vi "Create Contructor VIs.vi"   [LabVIEW 2015]
types:
  T1 = typedef "LVPositionTypeDef.ctl" = cluster{"Left":i32, "Top":i32}
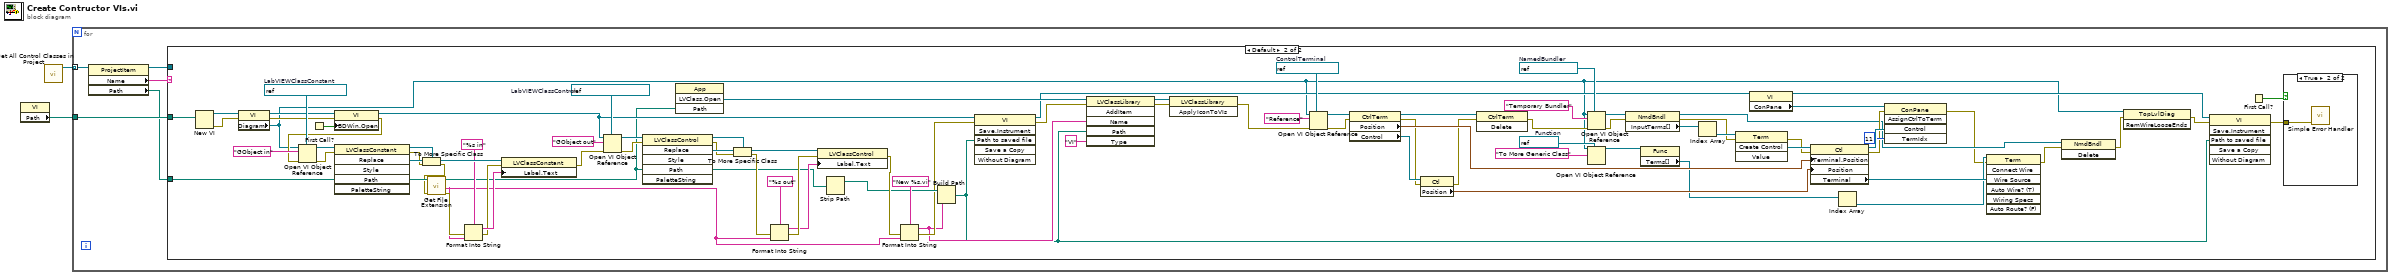
[diagram p0: block diagram]
diagram:
  n1 = property class="VI"() -> ("Path"=w1:path)  [unwired: 2 in, 2 out]
  n2 = call "Get All Control Classes in Project.vi"() -> ("All Control Classes"=w2:refnum<vi>[])  [unwired: 11 in]
  n3 = for {
    tunnel: w2 -> [w7] mode=indexing
    tunnel: w1 -> [w4]
    n4 = property class="ProjectItem"(reference=w7) -> (reference out=w5:refnum<vi>, "Name"=w6:string, "Path"=w3:path)  [unwired: 1 in, 1 out]
    n5 = case shown="Default" w6 {
      tunnel: w5 -> [_ _]
      tunnel: w4 -> [_ w96]
      tunnel: w3 -> [_ w79]
      frame "GObject.lvclass", "Generic.lvclass" {
      }
      frame Default {
        w18 = refnum<vi> refnum  # Function
        w43 = refnum<vi> refnum  # ControlTerminal
        w47 = refnum<vi> refnum  # NamedBundler
        w91 = refnum<vi> refnum  # LabVIEWClassControl
        w93 = refnum<vi> refnum  # LabVIEWClassConstant
        n6 = New VI(10:w96) -> (0:w86:errorcluster, 3:w95:refnum<vi>)  [unwired: 6 in]
        n7 = property class="VI"(reference=w95, error in=w86) -> (reference out=w85:refnum<vi>, error out=w84:errorcluster, "Diagram"=w10:refnum<vi>)
        n8 = First Call?() -> (First Call?: T/F=w22:bool)
        n9 = property class="VI"(reference=w85, error in=w84, "BDWin.Open"=w22) -> (reference out=w62:refnum<vi>, error out=w83:errorcluster)
        n10 = Open VI Object Reference(7:w93, 8:w83, 10:"GObject in" ("name/order"), 11:w10) -> (0:w87:errorcluster, 3:w92:refnum<vi>)
        n11 = invoke class="LVClassConstant" method="Replace"(reference=w92, error in=w87, "Path"=w79) -> (reference out=w80:refnum<vi>, error out=w74:errorcluster, "Replace"=w82:refnum<vi>)  [unwired: 3 in, 3 out]
        n12 = To More Specific Class(target class=w80, reference=w82, error in=w74) -> (specific class reference=w81:refnum<vi>, error out=w73:errorcluster)
        n13 = call <vilib>:"Get File Extension.vi"("error in (no error)"=w73, "file"=w79) -> ("error out"=w72:errorcluster, "filename without extension"=w59:string, "dup file"=w61:path)  [unwired: 5 in, 2 out]
        n14 = Format Into String(format string="%s in", error in=w72, w59) -> (resulting string=w77:string, error out=w71:errorcluster)  [unwired: 1 in]
        n15 = property class="LVClassConstant"(reference=w81, error in=w71, "Label.Text"=w77) -> (error out=w70:errorcluster)  [unwired: 1 out]
        n16 = Open VI Object Reference(7:w91, 8:w70, 10:"GObject out" ("name/order"), 11:w62) -> (0:w88:errorcluster, 3:w89:refnum<vi>)
        n17 = invoke class="LVClassControl" method="Replace"(reference=w89, error in=w88, "Path"=w61) -> (reference out=w75:refnum<vi>, error out=w69:errorcluster, "Replace"=w76:refnum<vi>)  [unwired: 3 in, 3 out]
        n18 = invoke class="App" method="LVClass.Open"("Path"=w61) -> ("LVClass.Open"=w63:refnum<vi>)  [unwired: 3 in, 3 out]
        n19 = To More Specific Class(target class=w75, reference=w76, error in=w69) -> (specific class reference=w66:refnum<vi>, error out=w68:errorcluster)
        n20 = Format Into String(format string="%s out", error in=w68, w59) -> (resulting string=w64:string, error out=w65:errorcluster)  [unwired: 1 in]
        n21 = property class="LVClassControl"(reference=w66, error in=w65, "Label.Text"=w64) -> (error out=w58:errorcluster)  [unwired: 1 out]
        n22 = Strip Path(path=w61) -> (stripped path=w57:path)  [unwired: 1 out]
        n23 = Format Into String(format string="New %s.vi", error in=w58, w59) -> (resulting string=w55:string, error out=w56:errorcluster)  [unwired: 1 in]
        n24 = Build Path(base path=w57, name or relative path=w55) -> (appended path=w50:path)
        n25 = invoke class="VI" method="Save.Instrument"(reference=w62, error in=w56, "Path to saved file"=w50) -> (reference out=w28:refnum<vi>, error out=w54:errorcluster)  [unwired: 3 in, 4 out]
        n26 = invoke class="LVClassLibrary" method="AddItem"(reference=w63, error in=w54, "Name"=w55, "Path"=w50, "Type"="VI") -> (reference out=w52:refnum<vi>, error out=w51:errorcluster)  [unwired: 1 in, 4 out]
        n27 = invoke class="LVClassLibrary" method="ApplyIconToVIs"(reference=w52, error in=w51) -> (error out=w42:errorcluster)  [unwired: 1 in, 2 out]
        n28 = Open VI Object Reference(7:w43, 8:w42, 10:"Reference" ("name/order"), 11:w10) -> (0:w40:errorcluster, 3:w41:refnum<vi>)
        n29 = property class="CtrlTerm"(reference=w41, error in=w40) -> (reference out=w35:refnum<vi>, error out=w31:errorcluster, "Position"=w33:T1, "Control"=w32:refnum<vi>)
        n30 = property class="Ctl"(reference=w32, error in=w31) -> (error out=w30:errorcluster, "Position"=w29:T1)  [unwired: 1 out]
        n31 = invoke class="CtrlTerm" method="Delete"(reference=w35, error in=w30) -> (error out=w34:errorcluster)  [unwired: 1 in, 2 out]
        n32 = Open VI Object Reference(7:w47, 8:w34, 10:"Temporary Bundler" ("name/order"), 11:w10) -> (0:w38:errorcluster, 3:w48:refnum<vi>)
        n33 = Open VI Object Reference(7:w18, 10:"To More Generic Class" ("name/order"), 11:w10) -> (3:w16:refnum<vi>)  [unwired: 1 in, 1 out]
        n34 = property class="NmdBndl"(reference=w48, error in=w38) -> (reference out=w13:refnum<vi>, error out=w37:errorcluster, "InputTerms[]"=w46:refnum<vi>[])
        n35 = property class="Func"(reference=w16) -> ("Terms[]"=w15:refnum<vi>[])  [unwired: 1 in, 2 out]
        n36 = Index Array(array=w46) -> (element=w45:refnum<vi>)  [unwired: 1 in]
        n37 = invoke class="Term" method="Create Control"(reference=w45, error in=w37) -> (error out=w36:errorcluster, "Create Control"=w39:refnum<vi>)  [unwired: 2 in, 2 out]
        n38 = property class="VI"(reference=w28) -> (reference out=w27:refnum<vi>, "ConPane"=w26:refnum<vi>)  [unwired: 1 in, 1 out]
        n39 = property class="Ctl"(reference=w39, error in=w36, "Terminal.Position"=w33, "Position"=w29) -> (reference out=w25:refnum<vi>, error out=w23:errorcluster, "Terminal"=w19:refnum<vi>)
        n40 = Index Array(array=w15) -> (element=w14:refnum<vi>)  [unwired: 1 in]
        n41 = invoke class="ConPane" method="AssignCtrlToTerm"(reference=w26, error in=w23, "Control"=w25, "TermIdx"=u32 11 ("Terminal Index")) -> (error out=w11:errorcluster)  [unwired: 1 in, 4 out]
        n42 = invoke class="Term" method="Connect Wire"(reference=w14, error in=w11, "Wire Source"=w19) -> (error out=w12:errorcluster)  [unwired: 4 in, 6 out]
        n43 = invoke class="NmdBndl" method="Delete"(reference=w13, error in=w12) -> (error out=w9:errorcluster)  [unwired: 1 in, 2 out]
        n44 = invoke class="TopLvlDiag" method="RemWireLooseEnds"(reference=w10, error in=w9) -> (error out=w8:errorcluster)  [unwired: 1 in, 2 out]
        n45 = invoke class="VI" method="Save.Instrument"(reference=w27, error in=w8, "Path to saved file"=w50) -> (error out=w21:errorcluster)  [unwired: 3 in, 5 out]
        n46 = First Call?() -> (First Call?: T/F=w20:bool)
        n47 = case shown="True" w20 {
          tunnel: w21 -> [_ w97]
          frame False {
          }
          frame True {
            n48 = call <vilib>:"Simple Error Handler.vi"("error in (no error)"=w97) -> ()  [unwired: 4 in, 5 out]
          }
        }
      }
    }
  }
